vi "SET_ELEVATOR_TARGET.vi"(10 "argv":string[](array[string]), 11 "args":u8) -> ()   [LabVIEW 2014]
uses:
  Robot Global Data.vi
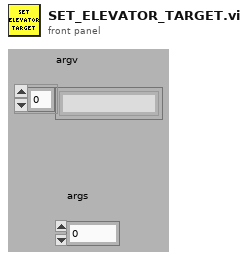
[diagram p1: front panel]
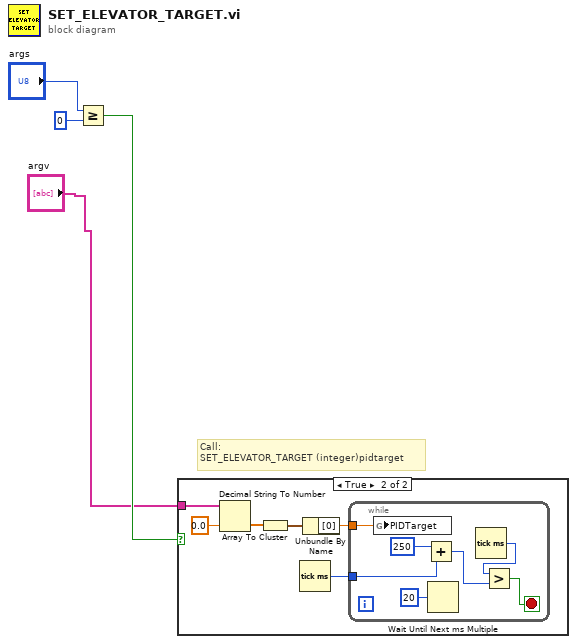
[diagram p0: block diagram]
diagram:
  # "Call:\nSET_ELEVATOR_TARGET (integer)pidtarget"
  n1 = Greater Or Equal?(x="args", y=u8 0) -> (x >= y?=w4:bool)
  n2 = case shown="True" w4 {
    tunnel: "argv" -> [_ w10]
    frame False {
    }
    frame True {
      n3 = Decimal String To Number(string=w10, default (0L)=0.0 ("default (0 I32)")) -> (number=w8:dbl[])  [unwired: 2 out]
      n4 = Array To Cluster(array=w8) -> (cluster=w7:cluster{"[0]":dbl, "[1]":dbl})
      n5 = Tick Count (ms)() -> (millisecond timer value=w5:u32)
      n6 = Unbundle By Name(w7) -> ("[0]"=w6:dbl)
      n7 = while {
        tunnel: w6 -> [w17]
        tunnel: w5 -> [w15]
        stop <- w14 stop-if-true
        n8 = global write "Robot Global Data.vi" "PIDTarget"(w17) -> ()
        n9 = Add(x=u32 250, y=w15) -> (x+y=w12:u32)
        n10 = Wait Until Next ms Multiple(millisecond multiple=u32 20) -> ()  [unwired: 1 out]
        n11 = Tick Count (ms)() -> (millisecond timer value=w11:u32)
        n12 = Greater?(x=w11, y=w12) -> (0:w14:bool)
      }
    }
  }
